vi "Eve_result_string.vi"(11 "Boolean array":bool[](array[boolean])) -> (3 "String":string)   [LabVIEW 2019]
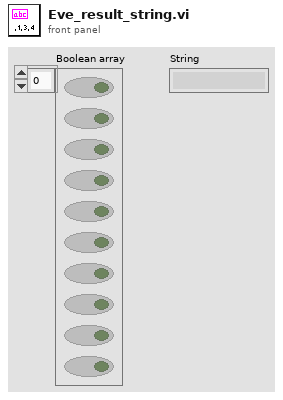
[diagram p1: front panel]
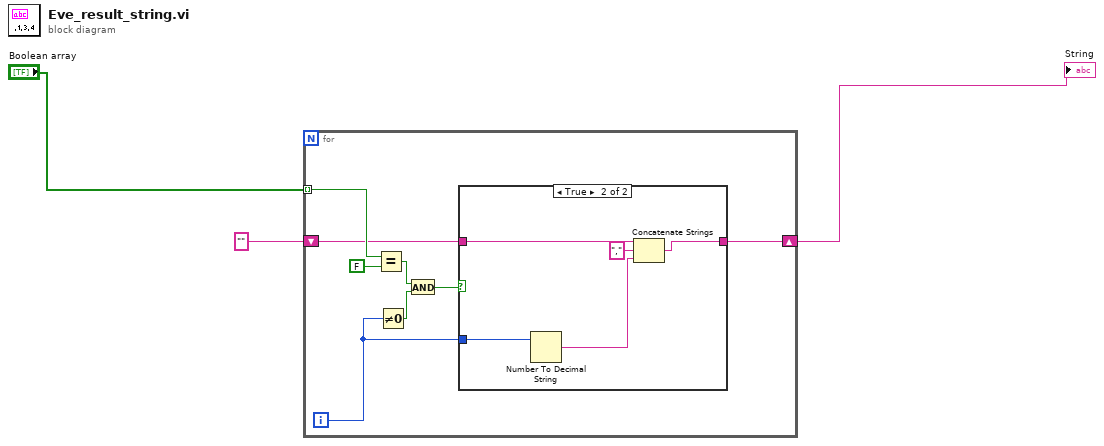
[diagram p0: block diagram]
diagram:
  n1 = for {
    tunnel: "Boolean array" -> [w11] mode=indexing
    shift-right: [w8] -> w3
    shift-left: "" -> [w9]
    i -> [w7]
    n2 = Equal?(x=w11, y=FALSE) -> (x = y?=w5:bool)
    n3 = Not Equal To 0?(x=w7) -> (x != 0?=w4:bool)
    n4 = And(x=w5, y=w4) -> (x .and. y?=w6:bool)
    n5 = case shown="True" w6 {
      tunnel: w7 -> [_ w17]
      tunnel: w9 -> [w12 w16]
      tunnel: [w12 w13] -> w8
      frame False {
      }
      frame True {
        n6 = Number To Decimal String(number=w17) -> (decimal integer string=w14:string)  [unwired: 1 in]
        n7 = Concatenate Strings(w16, "," ("string"), w14) -> (w13:string)
      }
    }
  }
  "String" <- w3
